vi "Maintenance.vi"() -> ()   [LabVIEW 2016, in "User Interface.lvlib"]
uses:
  User Interface.lvlib
  Maintenance command.ctl
  Database/Database.lvlib
  CAN/CAN.lvlib
  DAQ Hardware/DAQ Hardware.lvlib
  DAQ IO/DAQ IO.lvlib
  DC PWS/DC PWS.lvlib
  DMM/DMM.lvlib
  Func Generator/Func Generator.lvlib
  Oscilloscope/Oscilloscope.lvlib
  S-Matrix/S-Matrix.lvlib
  ARINC/ARINC.lvlib
  Maintenance Data highway.ctl
  Environment Chamber/Environment Chamber.lvlib
  VI Name.ctl
  CVT/CVT.lvlib
  DAQ Hardware/Timing AI DAQ Setting.ctl
  Instrument Address Command.ctl
  <vilib>/Utility/miscctls.llb/LVPointTypeDef.ctl
  Data Analysis/Data Analysis.lvlib
  Serial Hardware/Serial Hardware.lvlib
  <vilib>/NI/Current Value Table/Current Value Table.lvlib
  <vilib>/NI/Current Value Table/DataTypes/Boolean_Static Read.vi
  <vilib>/xnet/xnet.llb/XNET Frame Type CAN.ctl
  <vilib>/xnet/xnet.llb/XNET Frame CAN.ctl
panel:
  out "Analog Data":cluster{"DBL Array":dbl[]}[](graph)
  in  "Apply Command":bool
  out "Time 2":string="Authentication"
  in  "View Data":bool
  in  "Tab Control":T1(tab)
  in  "Channel Data":dbl[][](array[numeric])
  in  "DIO Apply Comm":bool
  in  "NI DAQ Command":enum16{"Acquire DI", "Stop DI"}(ring) caption="INPUT COMMAND"
  in  "NI DIO Connected":bool=TRUE
  in  "Sweep Spacing":enum16{"Linear", "Logarithmic"}(ring)
  in  "Unit (0: Vpp)":enum16{"Vpp", "Vrms", "dB"}(ring)
  in  "Sweep Time(Sec)":dbl step=0.05 format="%_4f"
  in  "Stop Freq(Hz)":dbl step=0.05 format="%_4f"
  in  "Start Freq(Hz)":dbl step=0.05 format="%_4f"
  in  "DC Offset (V)":dbl step=0.05 format="%_4f"
  in  "Amplitude":dbl step=0.05 format="%_4f"
  in  "Frequency(1000 Hz)":dbl step=0.05 format="%_4f"
  in  "Input Command":enum16{"Standad Waveform", "Frequency Sweep"}(ring)
  in  "FGen_Apply Command":bool
  in  "F.Gen Connected":bool=TRUE
  in  "Function":T2(ring)
  in  "Digital Output":T3
  in  "NI DAQ Control":T4={"NI DAQ Connected"=TRUE, "NI DAQ Command"=enum."Acquire AI", "AO Name"="AI 0", "AO Data In"=0.0, "Sampling rate"=5000.0, "Apply Command"=FALSE} {"Sampling rate" step=0.05; "AO Data In" step=0.05}
  in  "Digital Output":T5
  in  "DMM Control":T6={"DMM Connected"=TRUE, "Data Out"=0.0, "DMM Command"=enum."DC Voltage", "Apply Command"=FALSE, "Continuity"=FALSE} {"Data Out" step=0.05}
  out "Digital Input":T7
  out "Voltage(V)":dbl step=0.05 format="%2_4f"
  out "Current(A)":dbl step=0.05 format="%_4f"
  out "Data Out":dbl step=0.05
  in  "Data In":dbl step=0.05
  in  "DC Apply Command":bool
  in  "DC PWS Connected":bool=TRUE
  in  "DC PWS Command":T8(ring) caption="INPUT COMMAND"
  in  "Scope Apply Command":bool
  in  "Scope Channel":T9(ring) caption="Channel"
  in  "Scope Connected":bool=TRUE
  in  "Scope Command":T10(ring) caption="INPUT COMMAND"
  in  "Serial Command":T11(ring) caption="Measurement Command"
  in  "Serial Apply Command":bool
  in  "Command":string
  in  "Serial Connected":bool=TRUE
  out "CAN Monitor":string[][](table)
  in  "NI DAQ Connected":bool=TRUE
  in  "NI CAN Command":T12(ring)
  in  "Baud rate":dbl caption="Baudrate(Kbps)" step=0.05
  in  "CAN Command":bool
  in  "Interface Name":refnum<k21>
  in  "CAN Frame":T13[](array[typedef])=[{"timestamp"=timestamp(0 s since 1904-01-01), "payload"=[1, 2, 3, 4, 5, 6, 7, 8], "identifier"=2, "type"=0, "extended?"=FALSE, "echo?"=FALSE}, {"timestamp"=timestamp(0 s since 1904-01-01), "payload"=[0, 1, 2, 3, 4, 5, 6, 7], "identifier"=3, "type"=0, "extended?"=FALSE, "echo?"=FALSE}] {"payload" format="%x"; "timestamp" format="%<%.7X\n%x>T"; "type" items=["CAN Data"=0, "CAN Remote"=1, "CAN Bus Error"=2, "CAN 2.0 Data"=8, "CAN FD Data"=16, "CAN FD+BRS Data"=24, "J1939 Data"=192, "Delay"=224, "Log Trigger"=225, "Start Trigger"=226]; "identifier" format="%x"}
  out "CAN Monitor":string[][](table)
  out "Humidity":dbl step=0.05 format="%.2g"
  out "Temperature":dbl step=0.05 format="%.2g"
  out "Program State":T15 {"Remaining Counter B" step=0.05 format="%.2g"; "Remaining Counter A" step=0.05 format="%.2g"; "Remaining Time" step=0.05 format="%.2g"; "Humi Set Point" step=0.05 format="%.2g"; "Temp Set Point" step=0.05 format="%.2g"; "Step No" step=0.05 format="%.2g"; "Program No" step=0.05 format="%.2g"}
  in  "Meas Command":T16(ring) caption="Measurement Command"
  in  "ESPEC Apply Command":bool
  in  "ESPEC Connected":bool=TRUE
  in  "Exit":bool
  in  "DAQ Type":enum16{"Hardware", "Simulation"}(ring)=enum."Simulation"
  out "Fetch?":bool
  out "error out":errorcluster
  in  "error in (no error)":errorcluster
  # "NI CAN"
  # "NI 6363 DIO"
  # "NI 6515 Digital Input"
  # "NI 6515 Digital Output"
  # "Serial Inst Control"
  # "Scope Control"
  # "NI DIO(6515) Control"
  # "Function Generator Control"
  # "NI DAQ(6363) Control"
  # "DMM Control"
  # "DC Control"
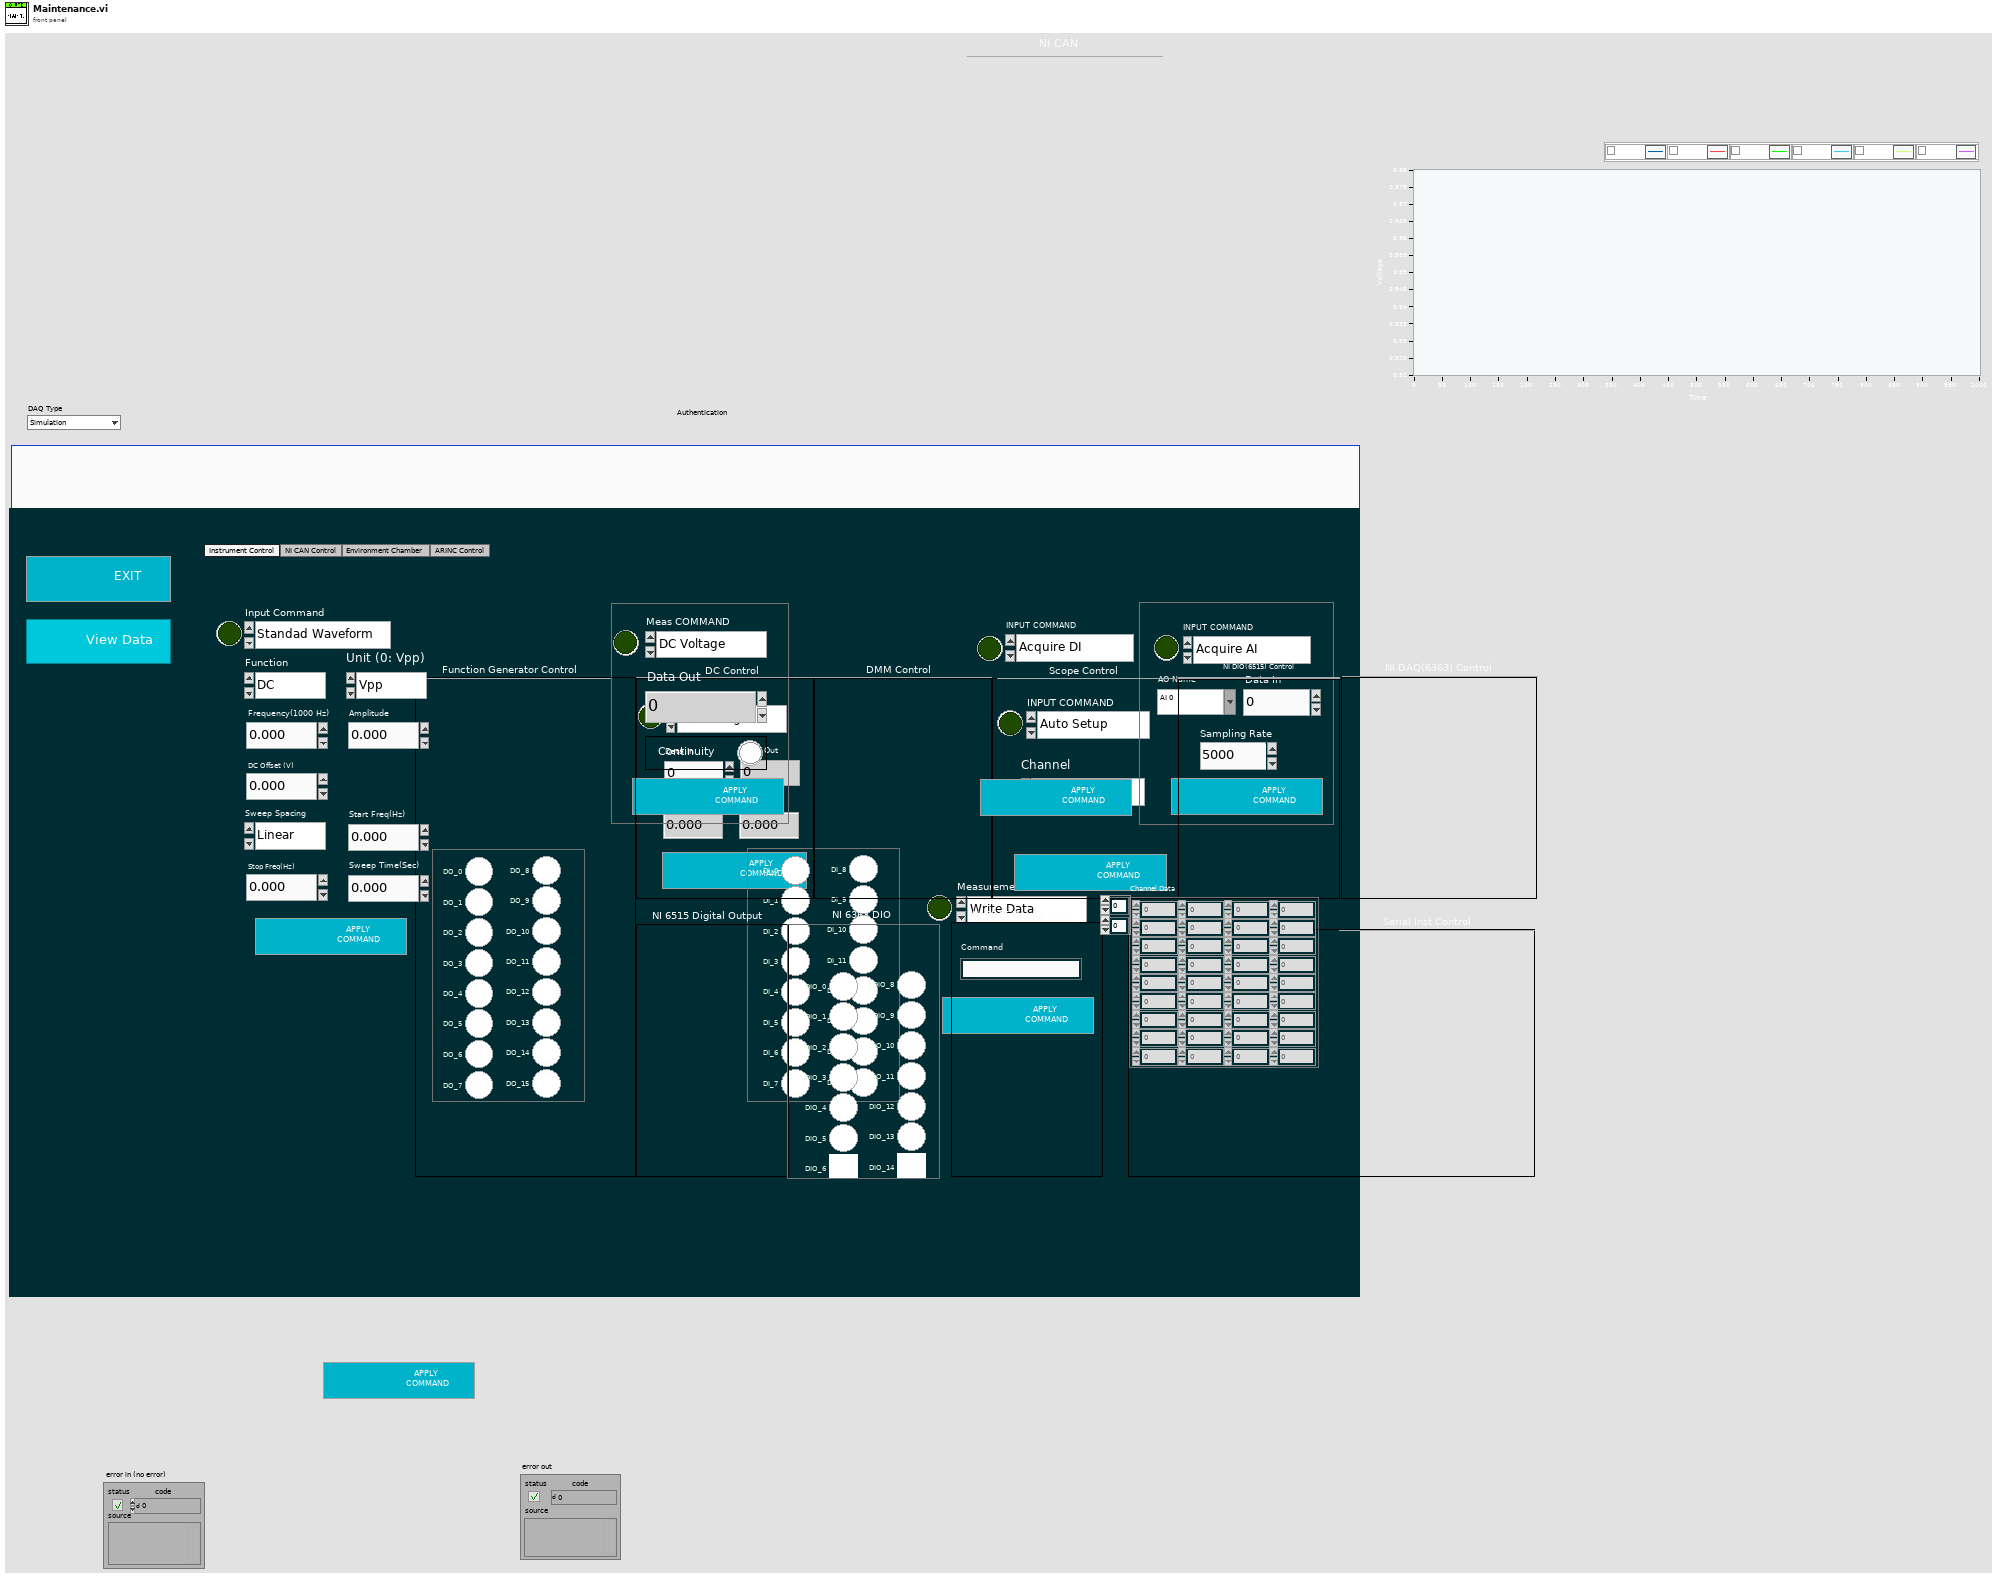
[diagram p1: front panel]
types:
  T1 = enum32{"Instrument Control", "NI CAN Control", "Environment Chamber", "ARINC Control"}
  T2 = enum16{"DC", "Sine", "Square", "Triangle", "Ramp", "Pulse", "Noise"}
  T3 = cluster{"DIO_0":bool, "DIO_1":bool, "DIO_2":bool, "DIO_3":bool, "DIO_4":bool, "DIO_5":bool, "DIO_6":bool, "DIO_7":bool, "DIO_8":bool, "DIO_9":bool, "DIO_10":bool, "DIO_11":bool, "DIO_12":bool, "DIO_13":bool, "DIO_14":bool, "DIO_15":bool}
  T4 = cluster{"NI DAQ Connected":bool, "NI DAQ Command":enum16{"Acquire AI", "Log Data", "Stop Log Data", "Stop AI", "Acquire DI", "Stop DI", "Update Rate", "Write AO"}, "AO Name":string, "AO Data In":dbl, "Sampling rate":dbl, "Apply Command":bool}
  T5 = cluster{"DO_0":bool, "DO_1":bool, "DO_2":bool, "DO_3":bool, "DO_4":bool, "DO_5":bool, "DO_6":bool, "DO_7":bool, "DO_8":bool, "DO_9":bool, "DO_10":bool, "DO_11":bool, "DO_12":bool, "DO_13":bool, "DO_14":bool, "DO_15":bool}
  T6 = cluster{"DMM Connected":bool, "Data Out":dbl, "DMM Command":enum16{"DC Voltage", "AC Voltage", "2 Wire Resistance", "Continuity"}, "Apply Command":bool, "Continuity":bool}
  T7 = cluster{"DI_0":bool, "DI_1":bool, "DI_2":bool, "DI_3":bool, "DI_4":bool, "DI_5":bool, "DI_6":bool, "DI_7":bool, "DI_8":bool, "DI_9":bool, "DI_10":bool, "DI_11":bool, "DI_12":bool, "DI_13":bool, "DI_14":bool, "DI_15":bool}
  T8 = enum16{"Set Voltage", "Set Current", "Set Power", "DC Parameter", "Measure Current", "Measure Voltage", "Output"}
  T9 = enum16{"Channel 1", "Channel 2", "Channel 3", "Channel 4"}
  T10 = enum16{"Auto Setup", "Config Channel", "Config DVM", "Acquire Waveform"}
  T11 = enum16{"Write Data", "Acquire Data", "Start Logging", "Stop Logging"}
  T12 = enum16{"Read CAN Data", "Write CAN Data", "Set Baudrate", "Start Logging Data", "Stop Logging Data"}
  T13 = typedef "XNET Frame CAN.ctl" = cluster{"timestamp":timestamp, "payload":u8[], "identifier":u32, "type":T14, "extended?":bool, "echo?":bool}
  T14 = typedef "XNET Frame Type CAN.ctl" = u8
  T15 = cluster{"Program No":dbl, "Step No":dbl, "Temp Set Point":dbl, "Humi Set Point":dbl, "Remaining Time":dbl, "Remaining Counter A":dbl, "Remaining Counter B":dbl}
  T16 = enum16{"Output On", "Output Off", "Acquire Data", "Start Log Data", "Stop Log Data", "Program Status"}
  T17 = typedef "LVPointTypeDef.ctl" = cluster{"Horizontal":i16, "Vertical":i16}
  T18 = typedef "User Interface.lvlib/Maintenance Data highway.ctl" = cluster{"Connection?":cluster{"DC PWS ?":bool, "DMM ?":bool, "FGEN ?":bool, "Oscill ?":bool, "NI DAQ ?":bool, "NI DIO ?":bool, "NI CAN ?":bool, "ESPEC ?":bool, "ARINC ?":bool, "MATRIX ?":bool}, "Inst Connected":refnum<vi>[], "Signal Name":cluster{"AI":string[], "AO":string[], "DI":string[], "DO":string[]}}
  T19 = typedef "User Interface.lvlib/Maintenance command.ctl" = enum16{"Init", "Main", "Close"}
  T20 = typedef "Current Value Table.lvlib/Group Data.ctl" = cluster{"Double":dbl[], "Single":sgl[], "I64":i64[], "I32":i32[], "I16":i16[], "I8":i8[], "U64":u64[], "U32":u32[], "U16":u16[], "U8":u8[], "String":string[], "Boolean":bool[], "Array of U8":cluster{"U8 Array":u8[]}[], "Array of U16":cluster{"U16 Array":u16[]}[], "Array of U32":cluster{"U32 Array":u32[]}[], "Array of U64":cluster{"U64 Array":u64[]}[], "Array of I64":cluster{"I64 Array":i64[]}[], "Array of I32":cluster{"I32 Array":i32[]}[], "Array of I16":cluster{"I16 Array":i16[]}[], "Array of I8":cluster{"I8 Array":i8[]}[], "Array of Double":cluster{"DBL Array":dbl[]}[], "Array of Single":cluster{"SGL Array":sgl[]}[], "Array of Boolean":cluster{"Boolean Array":bool[]}[], "Array of String":cluster{"String Array":string[]}[]}
  T21 = cluster{"Double[0]":dbl, "Double[1]":dbl, "Double[2]":dbl, "Double[3]":dbl, "Double[4]":dbl, "Double[5]":dbl, "Double[6]":dbl}
  T22 = cluster{"Boolean[0]":bool, "Boolean[1]":bool, "Boolean[2]":bool, "Boolean[3]":bool, "Boolean[4]":bool, "Boolean[5]":bool, "Boolean[6]":bool, "Boolean[7]":bool, "Boolean[8]":bool, "Boolean[9]":bool, "Boolean[10]":bool, "Boolean[11]":bool, "Boolean[12]":bool, "Boolean[13]":bool, "Boolean[14]":bool, "Boolean[15]":bool}
  T23 = typedef "User Interface.lvlib/Instrument Address Command.ctl" = enum16{"Init", "Read", "Write", "Close"}
  T24 = cluster{"Address":dbl, "Voltage Level":dbl, "Enable Output":bool}
  T25 = cluster{"Meas Command":enum16{"Voltage", "Current", "Power"}, "Address":dbl}
  T26 = cluster{"Waveform Function (1: Sine)":u16, "Frequency (1000 Hz)":dbl, "Amplitude (1)":dbl, "Unit (0: Vpp)":u16, "DC Offset (0.00 V)":dbl}
  T27 = cluster{"Sweep Spacing (0: Linear)":u16, "Sweep Time (1.00 s)":dbl, "Stop  Frequency (1000.0 Hz)":dbl, "Start Frequency (100.0 Hz)":dbl, "Enable/Disable Freq Sweep":bool}
  T28 = cluster{"Channel Name (0: Channel 1)":i32, "Coupling (1: DC)":i32, "Vertical Offset (0.0)":dbl, "Vertical Range (40.0 V)":dbl, "Probe Attenuation (1.0)":dbl, "Enable Channel (T: Enable)":bool, "Impedance (0: 1 MOhm)":i32, "Vertical Scale (5.0 V)":dbl, "Vertical Setting (1: Vertical Range)":i32}
  T29 = typedef "DAQ Hardware.lvlib/Timing AI DAQ Setting.ctl" = cluster{"rate":dbl, "samples per channel":i32, "sample mode":i32}
  T30 = typedef "User Interface.lvlib/VI Name.ctl" = enum16{"Dashboard", "Maintenance", "Recipe", "Inst Calibration", "Testing", "Report"}
  T31 = cluster{"[0]":bool, "[1]":bool, "[2]":bool, "[3]":bool, "[4]":bool, "[5]":bool, "[6]":bool, "[7]":bool, "[8]":bool, "[9]":bool}
  T32 = enum16{"DC Voltage", "AC Voltage", "2 Wire Resistance", "Continuity"}
  T33 = enum16{"Acquire AI", "Log Data", "Stop Log Data", "Stop AI", "Acquire DI", "Stop DI", "Update Rate", "Write AO"}
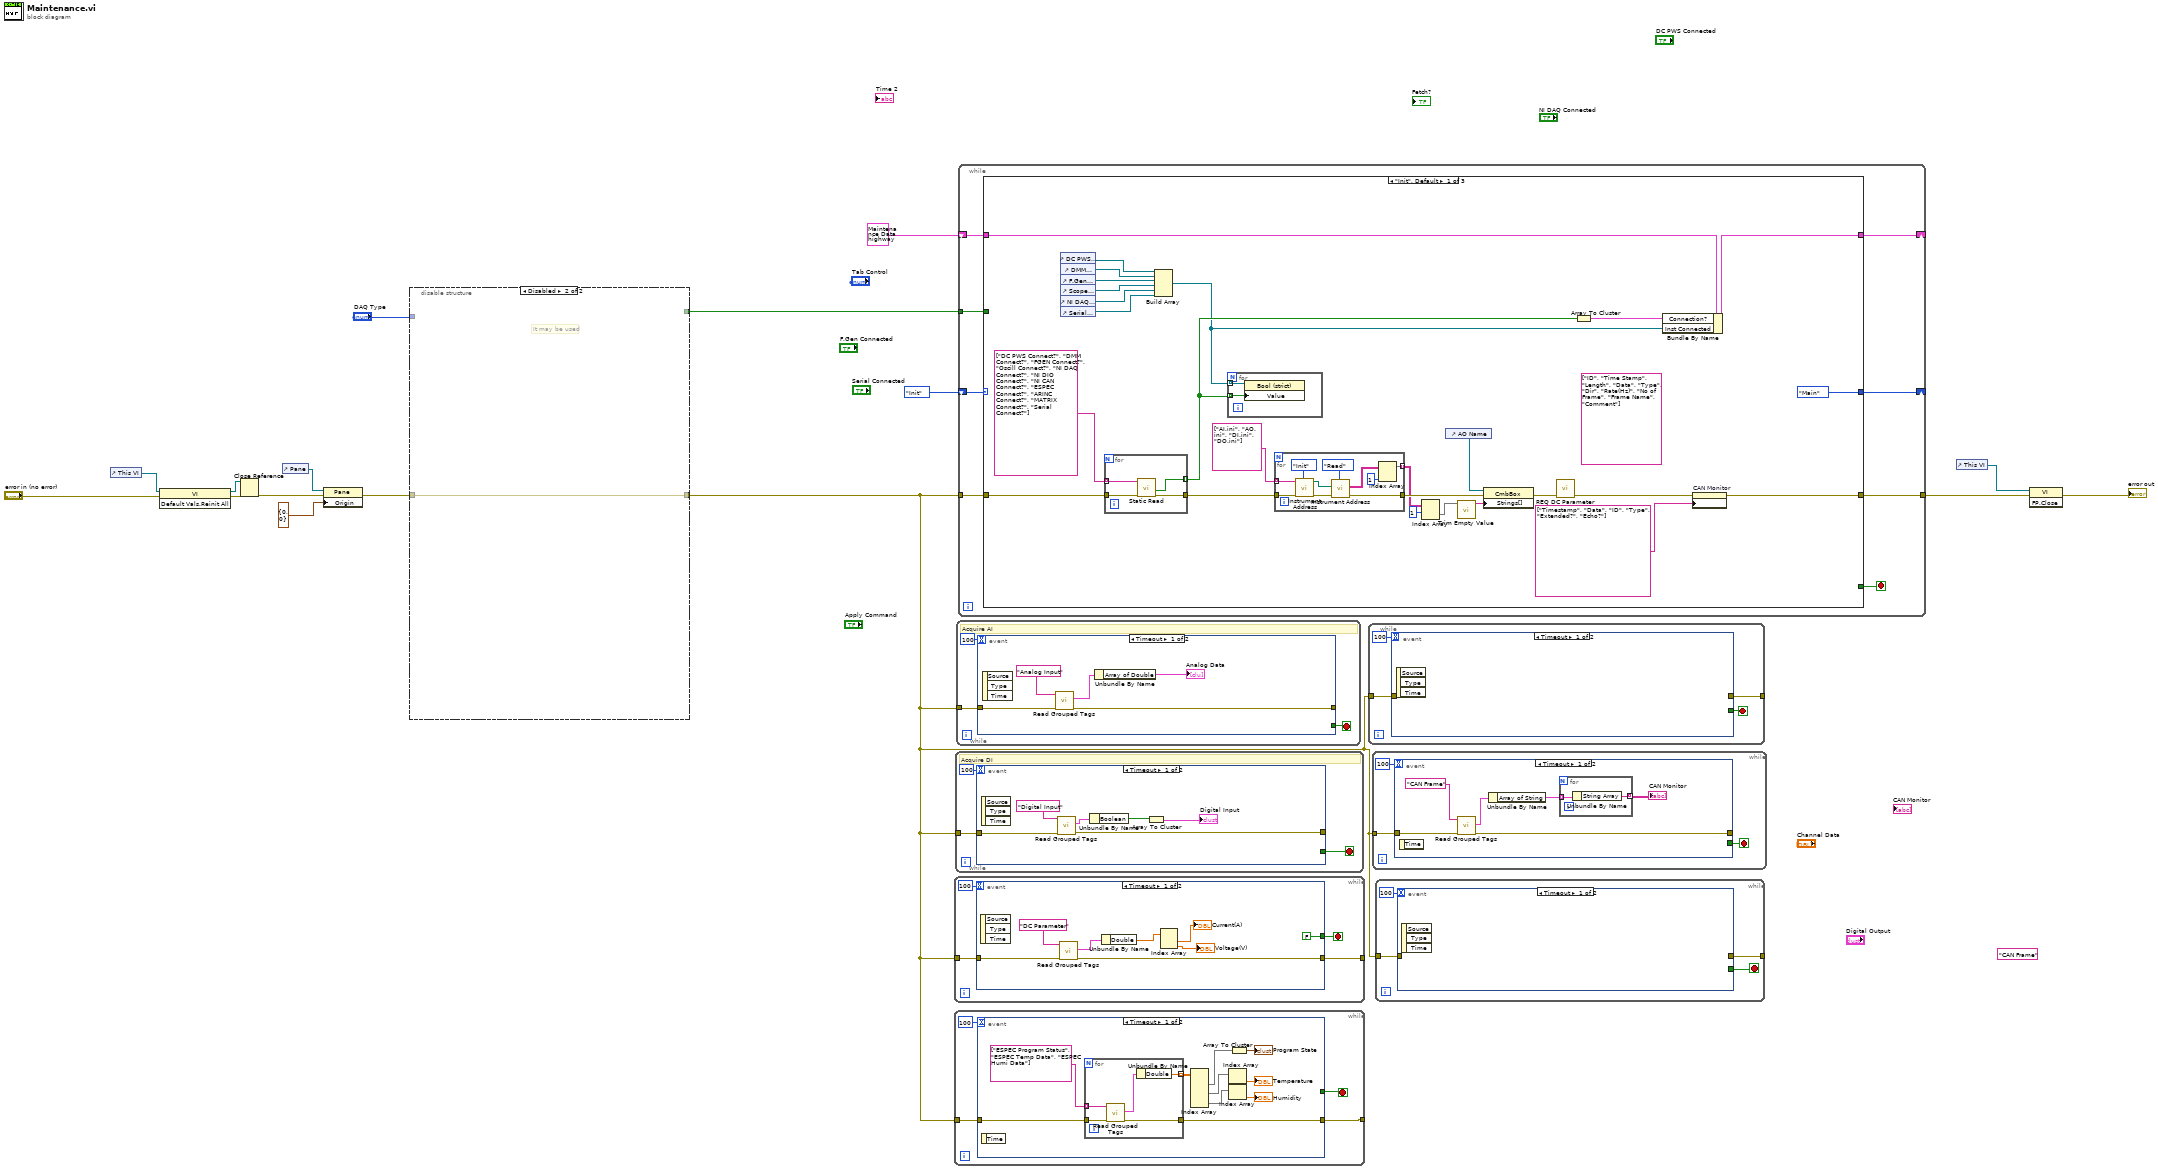
[diagram p0: block diagram]
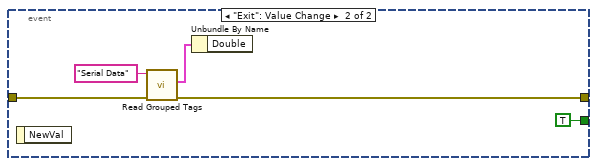
[diagram p2: hidden frame]
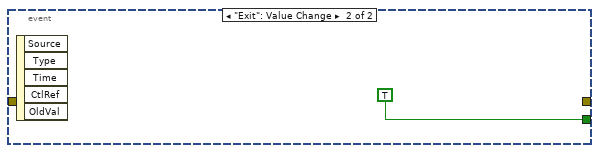
[diagram p3: hidden frame]
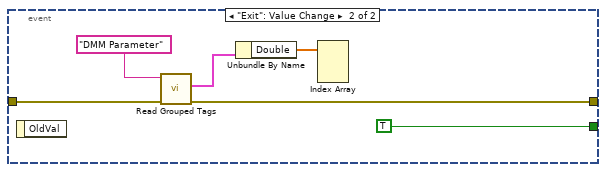
[diagram p4: hidden frame]
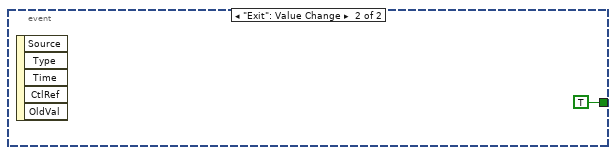
[diagram p5: hidden frame]
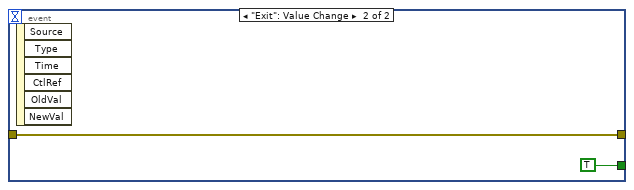
[diagram p6: hidden frame]
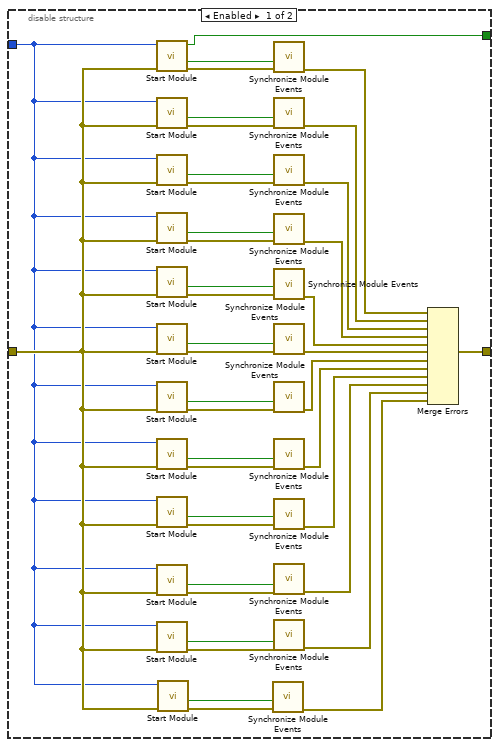
[diagram p7: hidden frame]
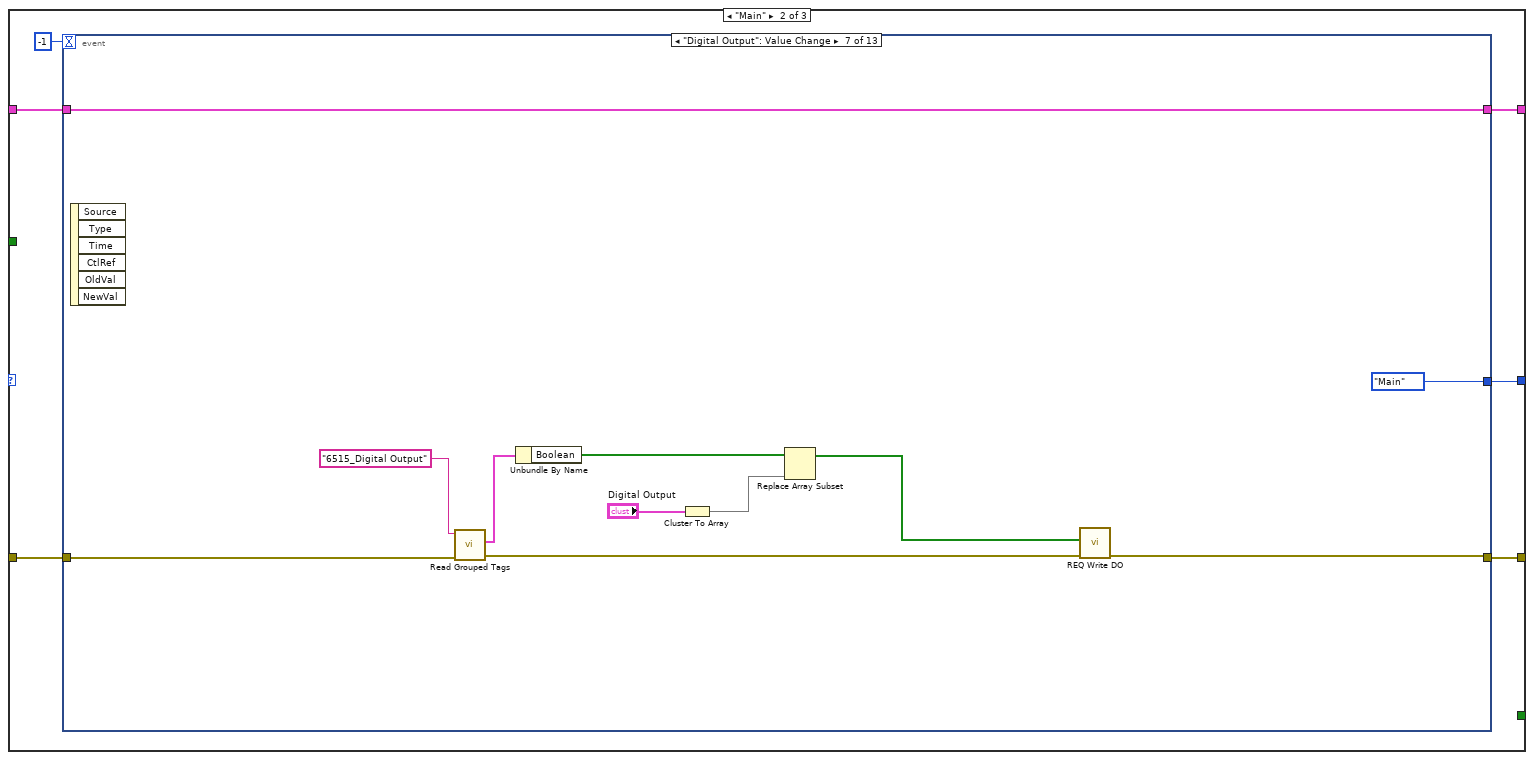
[diagram p8: hidden frame]
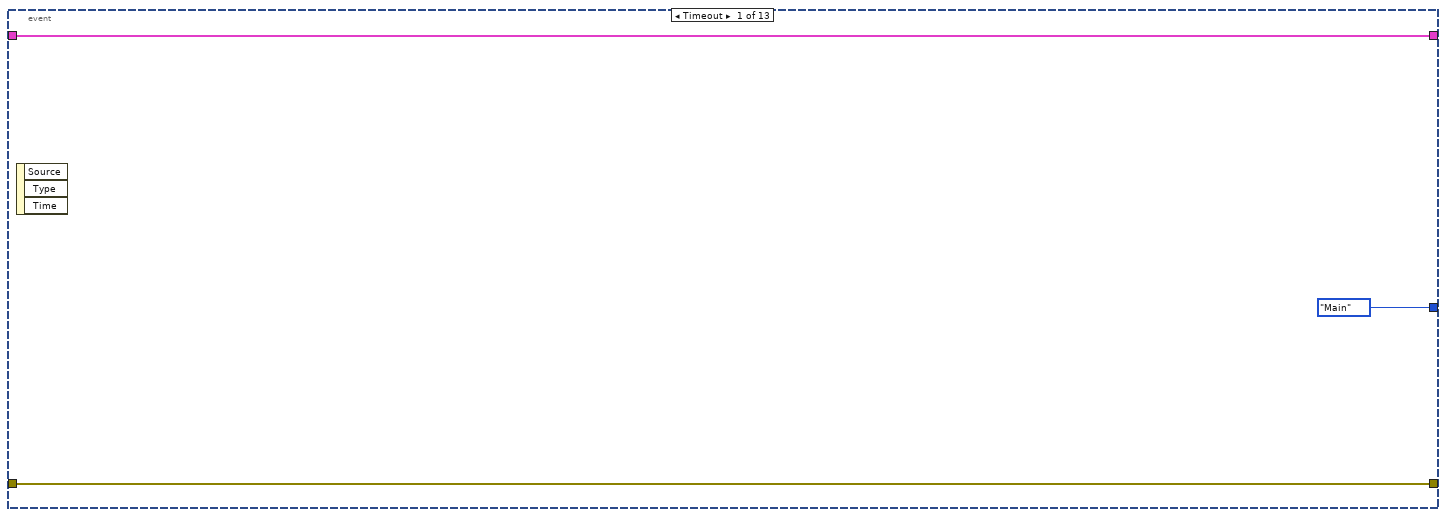
[diagram p9: hidden frame]
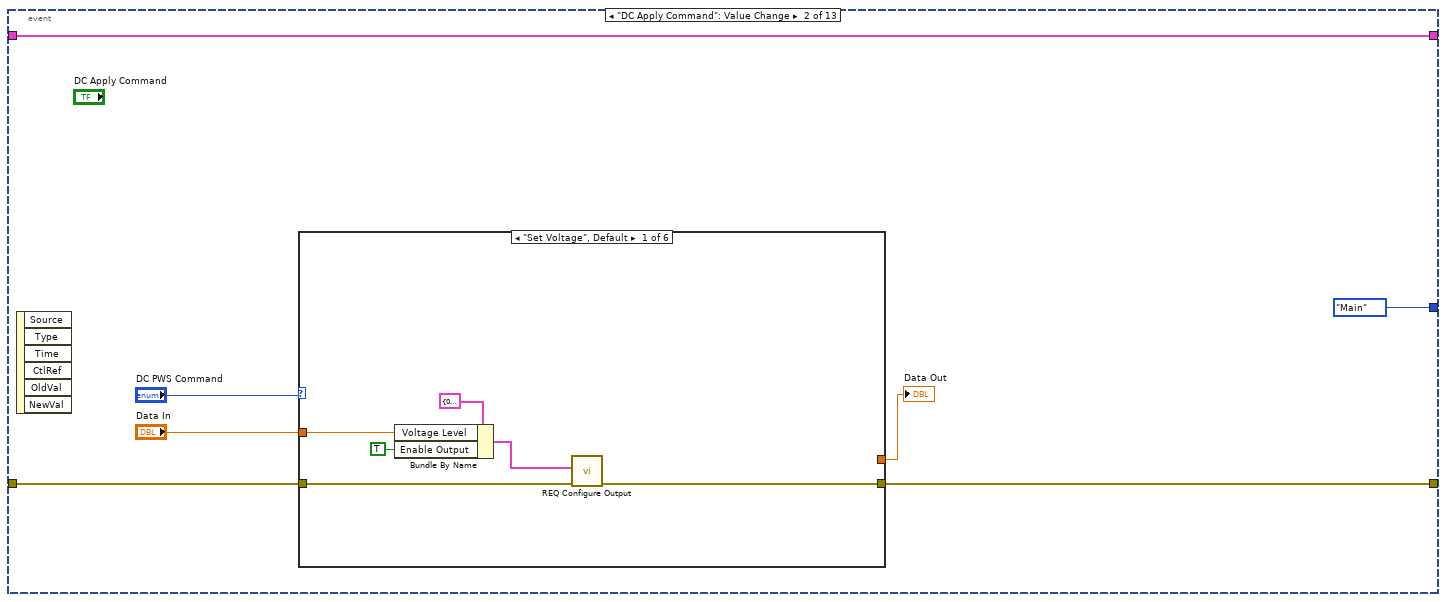
[diagram p10: hidden frame]
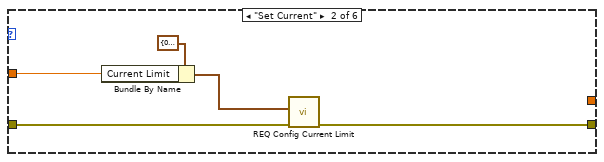
[diagram p11: hidden frame]
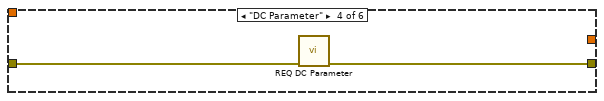
[diagram p13: hidden frame]
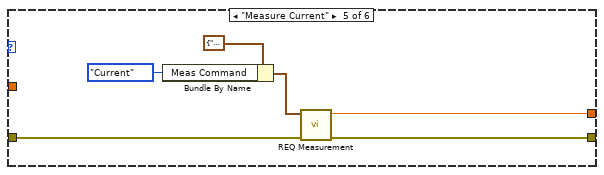
[diagram p14: hidden frame]
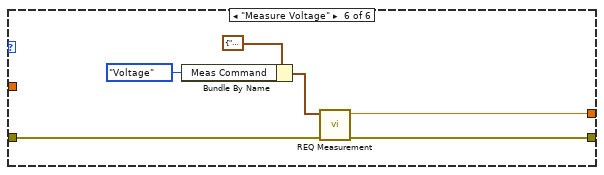
[diagram p15: hidden frame]
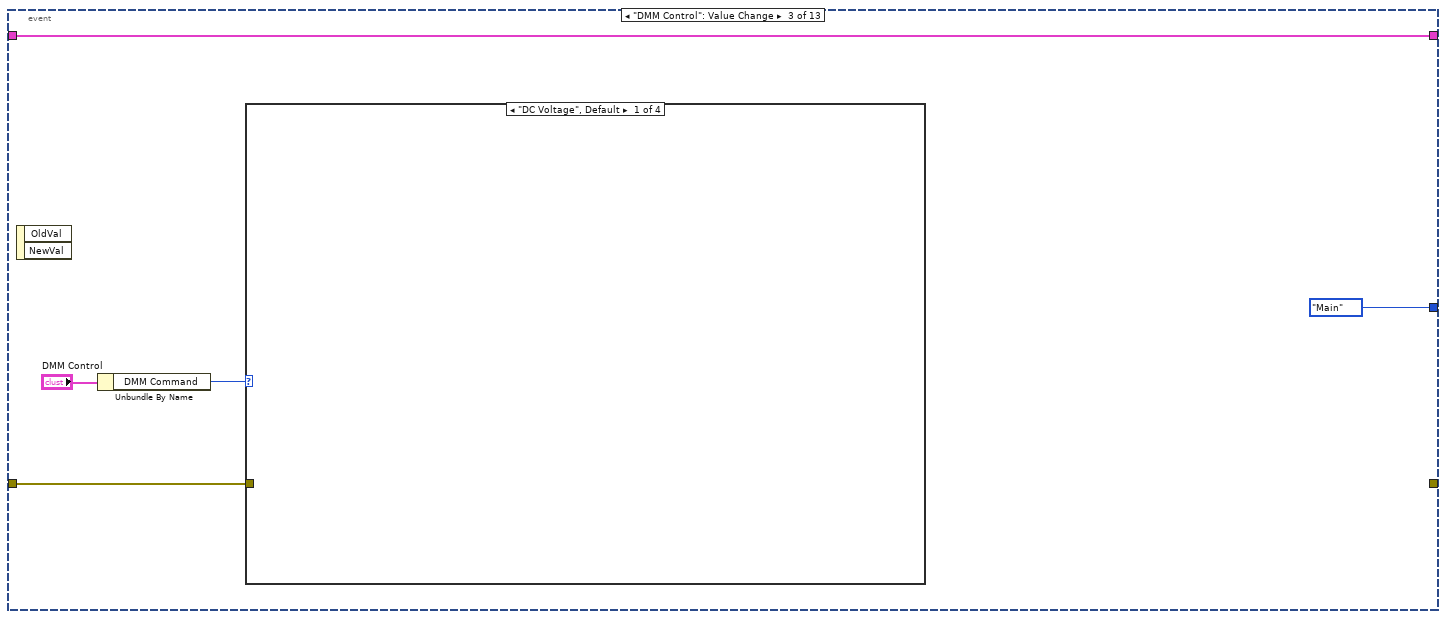
[diagram p16: hidden frame]
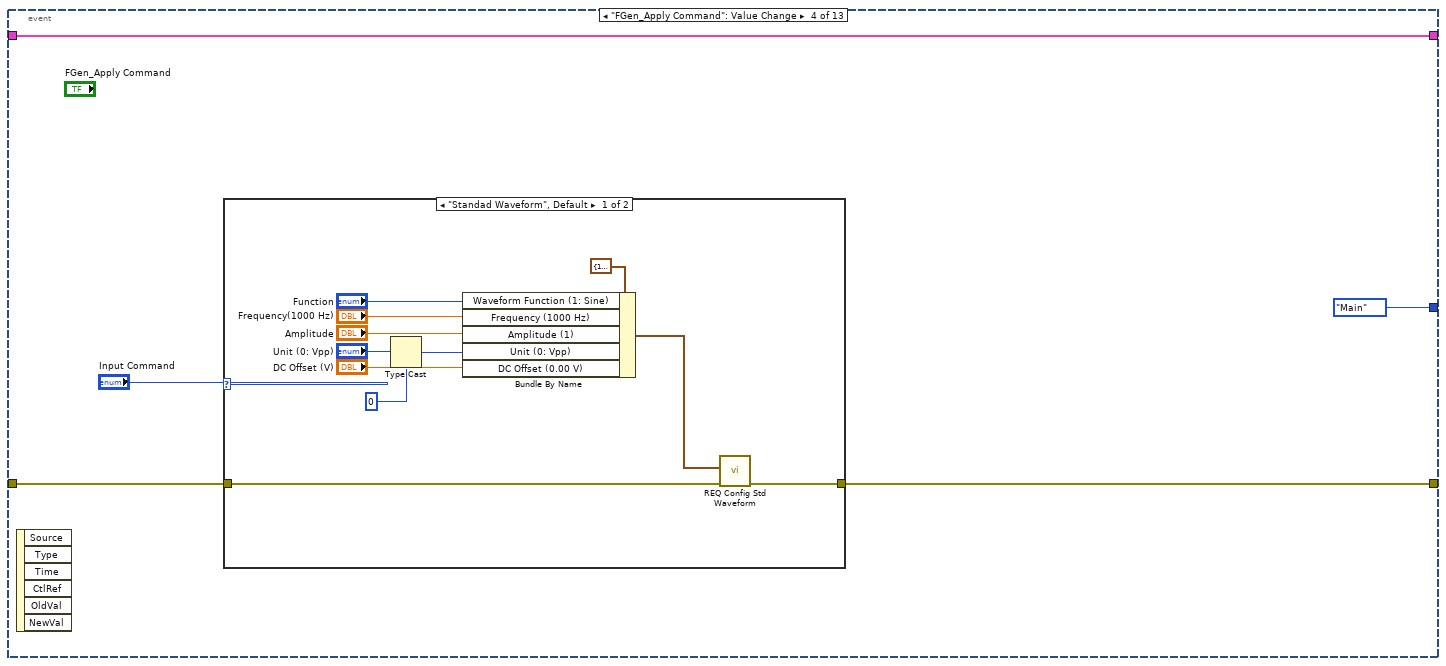
[diagram p20: hidden frame]
diagram:
  (unwired) "CAN Frame" ("Group")
  n1 = control-ref of="This VI"() -> (w12:refnum<vi>)
  n2 = invoke class="VI" method="Default Vals.Reinit All"(reference=w12, error in="error in (no error)") -> (reference out=w10:refnum<vi>, error out=w11:errorcluster)  [unwired: 1 in, 1 out]
  n3 = Close Reference(reference=w10, error in (no error)=w11) -> (error out=w9:errorcluster)
  n4 = control-ref of="Pane"() -> (w16:refnum<vi>)
  n5 = property class="Pane"(reference=w16, error in=w9, "Origin"=T17 {"Horizontal"=0, "Vertical"=0}) -> (error out=w4:errorcluster)  [unwired: 1 out]
  n6 = disable-structure shown="Disabled" {
    disable-tunnel: [w29 w57] -> w1
    disable-tunnel: [w28 _] -> w14
    disable-tunnel: w4 -> [w20 w57]
    disable-tunnel: "DAQ Type" -> [w19 _]
    frame Enabled {
      n7 = call "Start Module.vi"("error in"=w20, "DAQ Type"=w19) -> ("error out"=w23:errorcluster, "Wait for Event Sync?"=w22:bool, "Module Was Already Running?"=w28:bool)  [unwired: 6 in, 1 out]
      n8 = call "Start Module.vi"("error in"=w20, "DAQ Type"=w19) -> ("error out"=w49:errorcluster, "Wait for Event Sync?"=w47:bool)  [unwired: 6 in, 2 out]
      n9 = call "Start Module.vi"("error in"=w20, "DAQ Type"=w19) -> ("error out"=w50:errorcluster, "Wait for Event Sync?"=w46:bool)  [unwired: 6 in, 2 out]
      n10 = call "Start Module.vi"("error in"=w20, "DAQ Type"=w19) -> ("error out"=w48:errorcluster, "Wait for Event Sync?"=w45:bool)  [unwired: 6 in, 2 out]
      n11 = call "Start Module.vi"("error in"=w20, "DAQ Type"=w19) -> ("error out"=w51:errorcluster, "Wait for Event Sync?"=w44:bool)  [unwired: 6 in, 2 out]
      n12 = call "Start Module.vi"("error in"=w20, "DAQ Type"=w19) -> ("error out"=w52:errorcluster, "Wait for Event Sync?"=w43:bool)  [unwired: 6 in, 2 out]
      n13 = call "Start Module.vi"("error in"=w20, "DAQ Type"=w19) -> ("error out"=w53:errorcluster, "Wait for Event Sync?"=w42:bool)  [unwired: 6 in, 2 out]
      n14 = call "Start Module.vi"("error in"=w20, "DAQ Type"=w19) -> ("error out"=w54:errorcluster, "Wait for Event Sync?"=w41:bool)  [unwired: 6 in, 2 out]
      n15 = call "Start Module.vi"("error in"=w20, "DAQ Type"=w19) -> ("error out"=w55:errorcluster, "Wait for Event Sync?"=w40:bool)  [unwired: 6 in, 2 out]
      n16 = call "Start Module.vi"("error in"=w20, "DAQ Type"=w19) -> ("error out"=w56:errorcluster, "Wait for Event Sync?"=w39:bool)  [unwired: 6 in, 2 out]
      n17 = call "Start Module.vi"("error in"=w20, "DAQ Type"=w19) -> ("error out"=w26:errorcluster, "Wait for Event Sync?"=w25:bool)  [unwired: 6 in, 2 out]
      n18 = call "Start Module.vi"("error in"=w20, "DAQ Type"=w19) -> ("error out"=w21:errorcluster, "Wait for Event Sync?"=w18:bool)  [unwired: 6 in, 2 out]
      n19 = call "Synchronize Module Events.vi"("error in"=w21, "Wait for Event Sync?"=w18) -> ("error out"=w17:errorcluster)  [unwired: 9 in]
      n20 = call "Synchronize Module Events.vi"("error in"=w23, "Wait for Event Sync?"=w22) -> ("error out"=w38:errorcluster)  [unwired: 9 in]
      n21 = call "Synchronize Module Events.vi"("error in"=w49, "Wait for Event Sync?"=w47) -> ("error out"=w37:errorcluster)  [unwired: 9 in]
      n22 = call "Synchronize Module Events.vi"("error in"=w50, "Wait for Event Sync?"=w46) -> ("error out"=w36:errorcluster)  [unwired: 9 in]
      n23 = call "Synchronize Module Events.vi"("error in"=w48, "Wait for Event Sync?"=w45) -> ("error out"=w27:errorcluster)  [unwired: 9 in]
      n24 = call "Synchronize Module Events.vi"("error in"=w51, "Wait for Event Sync?"=w44) -> ("error out"=w35:errorcluster)  [unwired: 9 in]
      n25 = call "Synchronize Module Events.vi"("error in"=w52, "Wait for Event Sync?"=w43) -> ("error out"=w34:errorcluster)  [unwired: 9 in]
      n26 = call "Synchronize Module Events.vi"("error in"=w53, "Wait for Event Sync?"=w42) -> ("error out"=w33:errorcluster)  [unwired: 9 in]
      n27 = call "Synchronize Module Events.vi"("error in"=w54, "Wait for Event Sync?"=w41) -> ("error out"=w32:errorcluster)  [unwired: 9 in]
      n28 = call "Synchronize Module Events.vi"("error in"=w55, "Wait for Event Sync?"=w40) -> ("error out"=w31:errorcluster)  [unwired: 9 in]
      n29 = call "Synchronize Module Events.vi"("error in"=w56, "Wait for Event Sync?"=w39) -> ("error out"=w30:errorcluster)  [unwired: 9 in]
      n30 = call "Synchronize Module Events.vi"("error in"=w26, "Wait for Event Sync?"=w25) -> ("error out"=w24:errorcluster)  [unwired: 9 in]
      n31 = Merge Errors(w38, w37, w36, w27, w35, w34, w33, w32, w31, w30, w24, w17) -> (w29:errorcluster)
    }
    frame Disabled {
      # "It may be used"
    }
  }
  n32 = while {
    tunnel: w1 -> [w60]
    tunnel: [w59] -> _
    stop <- w61 stop-if-true
    n33 = event shown="[0] Timeout" {
      selector: _ -> [_ _]
      dyn-events: _ -> [_ _]
      timeout: 100 -> [_ _]
      tunnel: [FALSE TRUE] -> w61
      tunnel: w60 -> [w66 w70]
      tunnel: [w62 w70] -> w59
      event Timeout {
        n34 = event-data() -> ()  [unwired: 1 in, 3 out]
        n35 = call <vilib>:"Read Grouped Tags.vi"("error in (no error)"=w66, "Group"="DC Parameter") -> ("error out"=w62:errorcluster, "Data"=w67:T20)  [unwired: 8 in]
        n36 = Unbundle By Name(w67) -> ("Double"=w65:dbl[])
        n37 = Index Array(array=w65) -> (element #1=→"Current(A)":dbl, element #2=→"Voltage(V)":dbl)  [unwired: 2 in]
      }
      event "Exit": Value Change {
        n38 = event-data() -> ()  [unwired: 1 in, 1 out]
      }
    }
  }
  n39 = while {
    tunnel: w1 -> [w73]
    tunnel: [w72] -> _
    stop <- w75 stop-if-true
    n40 = event shown="[0] Timeout" {
      selector: _ -> [_ _]
      dyn-events: _ -> [_ _]
      timeout: 100 -> [_ _]
      tunnel: [_ TRUE] -> w75
      tunnel: w73 -> [w85 _]
      tunnel: [w84 _] -> w72
      event Timeout {
        n41 = event-data() -> ()  [unwired: 1 in, 1 out]
        n42 = for {
          tunnel: w85 -> [w90]
          tunnel: [w89] -> w84
          tunnel: string[] ["ESPEC Program Status", "ESPEC Temp Data", "ESPEC Humi Data"] -> [w88] mode=indexing
          tunnel: [w86] -> w81 mode=indexing
          n43 = call <vilib>:"Read Grouped Tags.vi"("error in (no error)"=w90, "Group"=w88) -> ("error out"=w89:errorcluster, "Data"=w87:T20)  [unwired: 8 in]
          n44 = Unbundle By Name(w87) -> ("Double"=w86:dbl[])
        }
        n45 = Index Array(array=w81) -> (element #1=w80:dbl[], element #2=w79:dbl[], element #3=w78:dbl[])  [unwired: 6 in]
        n46 = Index Array(array=w79) -> (element=→"Temperature":dbl)  [unwired: 1 in]
        n47 = Index Array(array=w78) -> (element=→"Humidity":dbl)  [unwired: 1 in]
        n48 = Array To Cluster(array=w80) -> (cluster=→"Program State":T21)
      }
      event "Exit": Value Change {
        n49 = event-data() -> ()  [unwired: 1 in, 5 out]
      }
    }
  }
  n50 = while {
    tunnel: w1 -> [w94]
    stop <- w92 stop-if-true
    # "Acquire DI"
    n51 = event shown="[0] Timeout" {
      selector: _ -> [_ _]
      dyn-events: _ -> [_ _]
      timeout: 100 -> [_ _]
      tunnel: w94 -> [w99 w101]
      tunnel: [w96 w101] -> _
      tunnel: [_ TRUE] -> w92
      event Timeout {
        n52 = event-data() -> ()  [unwired: 1 in, 3 out]
        n53 = call <vilib>:"Read Grouped Tags.vi"("error in (no error)"=w99, "Group"="Digital Input") -> ("error out"=w96:errorcluster, "Data"=w98:T20)  [unwired: 8 in]
        n54 = Unbundle By Name(w98) -> ("Boolean"=w97:bool[])
        n55 = Array To Cluster(array=w97) -> (cluster=→"Digital Input":T22)
      }
      event "Exit": Value Change {
        n56 = event-data() -> ()  [unwired: 1 in, 6 out]
      }
    }
  }
  n57 = while {
    tunnel: w1 -> [w103]
    stop <- w105 stop-if-true
    # "Acquire AI"
    n58 = event shown="[0] Timeout" {
      selector: _ -> [_ _]
      dyn-events: _ -> [_ _]
      timeout: 100 -> [_ _]
      tunnel: [_ TRUE] -> w105
      tunnel: w103 -> [w108 w111]
      tunnel: [w107 w111] -> _
      event Timeout {
        n59 = event-data() -> ()  [unwired: 1 in, 3 out]
        n60 = call <vilib>:"Read Grouped Tags.vi"("error in (no error)"=w108, "Group"="Analog Input") -> ("error out"=w107:errorcluster, "Data"=w110:T20)  [unwired: 8 in]
        n61 = Unbundle By Name(w110) -> ("Array of Double"=→"Analog Data":cluster{"DBL Array":dbl[]}[])
      }
      event "Exit": Value Change {
        n62 = event-data() -> ()  [unwired: 1 in, 6 out]
      }
    }
  }
  n63 = while {
    shift-right: [w118] -> _
    shift-left: Maintenance_command."Init" -> [w120]
    tunnel: w1 -> [w119]
    tunnel: w14 -> [w116]
    shift-right: [w114] -> _
    shift-left: T18 {"Connection?"={"DC PWS ?"=FALSE, "DMM ?"=FALSE, "FGEN ?"=FALSE, "Oscill ?"=FALSE, "NI DAQ ?"=FALSE, "NI DIO ?"=FALSE, "NI CAN ?"=FALSE, "ESPEC ?"=FALSE, "ARINC ?"=FALSE, "MATRIX ?"=FALSE}, "Inst Connected"=[], "Signal Name"={"AI"=[], "AO"=[], "DI"=[], "DO"=[]}} -> [w115]
    tunnel: [w113] -> w5
    stop <- w117 stop-if-true
    n64 = case shown="\"Init\", Default" w120 {
      tunnel: w119 -> [w143 w167 w383]
      tunnel: [Maintenance_command."Main" w164 Maintenance_command."Close"] -> w118
      tunnel: [_ _ TRUE] -> w117
      tunnel: w116 -> [_ _ w382]
      tunnel: w115 -> [w145 w166 w384]
      tunnel: [w142 w165 w384] -> w114
      tunnel: [w122 w163 w376] -> w113
      frame "Init", Default {
        (unwired) string[] ["ID", "Time Stamp", "Length", "Data", "Type", "Dir", "Rate(Hz)", "No of Frame", "Frame Name", "Comment"] ("Row Header Strings[]")
        n65 = control-ref of="DC PWS Connected"() -> (w140:refnum<vi>)
        n66 = control-ref of="DMM Connected"() -> (w139:refnum<vi>)
        n67 = control-ref of="F.Gen Connected"() -> (w138:refnum<vi>)
        n68 = control-ref of="Scope Connected"() -> (w137:refnum<vi>)
        n69 = control-ref of="NI DAQ Connected"() -> (w136:refnum<vi>)
        n70 = control-ref of="Serial Connected"() -> (w121:refnum<vi>)
        n71 = for {
          tunnel: string[] ["DC PWS Connect?", "DMM Connect?", "FGEN Connect?", "Oscill Connect?", "NI DAQ Connect?", "NI DIO Connect?", "NI CAN Connect?", "ESPEC Connect?", "ARINC Connect?", "MATRIX Connect?", "Serial Connect?"] -> [w162] mode=indexing
          tunnel: [w161] -> w135 mode=indexing
          tunnel: w143 -> [w160]
          tunnel: [w159] -> w134
          n72 = call-poly <vilib>:"Static Read.vi"("error in (no error)"=w160, "Tag Name"=w162) -> ("error out"=w159:errorcluster, "Value"=w161:bool)  [unwired: 8 in]
        }
        n73 = Build Array(w140, w139, w138, w137, w136, w121) -> (w125:refnum<vi>[])
        n74 = for {
          tunnel: w125 -> [w158] mode=indexing
          tunnel: w135 -> [w157] mode=indexing
          n75 = property class="Bool (strict)"(reference=w158, "Value"=w157) -> ()  [unwired: 1 in, 2 out]
        }
        n76 = for {
          tunnel: w134 -> [w154]
          tunnel: string[] ["AI.ini", "AO.ini", "DI.ini", "DO.ini"] -> [w151] mode=indexing
          tunnel: [w148] -> w130 mode=indexing
          tunnel: [w147] -> w132
          n77 = call "Instrument Address.vi"("Command"=Instrument_Address_Command."Init", "error in (no error)"=w154, "name or relative path"=w151) -> ("error out"=w153:errorcluster, "path_out"=w152:path)  [unwired: 6 in, 1 out]
          n78 = call "Instrument Address.vi"("Command"=Instrument_Address_Command."Read", "error in (no error)"=w153, "path_in"=w152) -> ("error out"=w147:errorcluster, "Instrument Parameter"=w150:string[][])  [unwired: 6 in, 1 out]
          n79 = Index Array(array=w150, index (col)=1 ("disabled index (col)")) -> (element=w148:string[])  [unwired: 1 in]
        }
        n80 = Index Array(array=w130, index (row)=1) -> (element=w129:string[])  [unwired: 1 in]
        n81 = control-ref of="AO Name"() -> (w131:refnum<vi>)
        n82 = call "Trim Empty Value.vi"("Data In"=w129) -> ("Data Out"=w128:string[])  [unwired: 10 in]
        n83 = property class="CmbBox"(reference=w131, error in=w132, "Strings[]"=w128) -> (error out=w126:errorcluster)  [unwired: 1 out]
        n84 = call "REQ DC Parameter.vi"("error in"=w126) -> ("error out"=w124:errorcluster)  [unwired: 10 in]
        n85 = Array To Cluster(array=w135) -> (cluster=w141:T31)
        n86 = Bundle By Name(cluster=w145, "Connection?"=w141, "Inst Connected"=w125) -> (w142:T18)
        n87 = property on="CAN Monitor" class="Tbl (strict)"(error in=w124, "Column Headers[]"=string[] ["Timestamp", "Data", "ID", "Type", "Extended?", "Echo?"]) -> (error out=w122:errorcluster)  [unwired: 1 in, 1 out]
      }
      frame "Main" {
        n88 = event shown="[6] \"Digital Output\": Value Change" {
          selector: _ -> [_ _ _ _ _ _ _ _ _ _ _ _ _]
          dyn-events: _ -> [_ _ _ _ _ _ _ _ _ _ _ _ _]
          timeout: -1 -> [_ _ _ _ _ _ _ _ _ _ _ _ _]
          tunnel: w167 -> [w170 w177 w206 w212 w239 w258 w277 w288 w325 w333 w342 w358 w374]
          tunnel: w166 -> [w169 w178 w209 w214 w241 w260 w282 w291 w327 w331 w344 w361 w373]
          tunnel: [w169 w178 w209 w214 w241 w260 w282 w291 w327 w331 w344 w361 w373] -> w165
          tunnel: [Maintenance_command."Main" Maintenance_command."Main" Maintenance_command."Main" Maintenance_command."Main" Maintenance_command."Main" Maintenance_command."Main" Maintenance_command."Main" Maintenance_command."Main" Maintenance_command."Main" Maintenance_command."Main" Maintenance_command."Main" Maintenance_command."Main" Maintenance_command."Close"] -> w164
          tunnel: [w170 w175 _ w211 w238 w257 w272 w287 w322 w332 w340 w357 w374] -> w163
          event Timeout {
            n89 = event-data() -> ()  [unwired: 1 in, 3 out]
          }
          event "DC Apply Command": Value Change {
            n90 = event-data() -> ()  [unwired: 1 in, 6 out]
            n91 = case shown="\"Set Voltage\", Default" "DC PWS Command" {
              tunnel: w177 -> [w184 w189 w190 w192 w195 w204]
              tunnel: [w181 w188 w190 w191 w194 w200] -> w175
              tunnel: "Data In" -> [w180 w187 _ _ _ _]
              tunnel: [_ _ _ _ w193 w199] -> w172
              frame "Set Voltage", Default {
                n92 = Bundle By Name(cluster=T24 {"Address"=0.0, "Voltage Level"=0.0, "Enable Output"=FALSE} ("Output Setting"), "Voltage Level"=w180, "Enable Output"=TRUE) -> (w182:T24)
                n93 = call "REQ Configure Output.vi"("error in"=w184, "Output Setting"=w182) -> ("error out"=w181:errorcluster)  [unwired: 9 in]
              }
              frame "Set Current" {
                n94 = Bundle By Name(cluster=cluster{"Address":dbl, "Current Limit":dbl} {"Address"=0.0, "Current Limit"=0.0} ("Current Limit Setting"), "Current Limit"=w187) -> (w185:cluster{"Address":dbl, "Current Limit":dbl})
                n95 = call "REQ Config Current Limit.vi"("error in"=w189, "Current Limit Setting"=w185) -> ("error out"=w188:errorcluster)  [unwired: 9 in]
              }
              frame "Set Power" {
              }
              frame "DC Parameter" {
                n96 = call "REQ DC Parameter.vi"("error in"=w192) -> ("error out"=w191:errorcluster)  [unwired: 10 in]
              }
              frame "Measure Current" {
                n97 = Bundle By Name(cluster=T25 {"Meas Command"=enum."Voltage", "Address"=0.0} ("Meas Parameter"), "Meas Command"=enum16{"Voltage", "Current", "Power"}."Current") -> (w197:T25)
                n98 = call "REQ Measurement.vi"("error in"=w195, "Meas Parameter"=w197) -> ("error out"=w194:errorcluster, "Value"=w193:dbl)  [unwired: 7 in, 1 out]
              }
              frame "Measure Voltage" {
                n99 = Bundle By Name(cluster=T25 {"Meas Command"=enum."Voltage", "Address"=0.0} ("Meas Parameter"), "Meas Command"=enum16{"Voltage", "Current", "Power"}."Voltage") -> (w202:T25)
                n100 = call "REQ Measurement.vi"("error in"=w204, "Meas Parameter"=w202) -> ("error out"=w200:errorcluster, "Value"=w199:dbl)  [unwired: 7 in, 1 out]
              }
            }
            "Data Out" <- w172
          }
          event "DMM Control": Value Change {
            n101 = event-data() -> ()  [unwired: 1 in, 2 out]
            n102 = Unbundle By Name("DMM Control") -> ("DMM Command"=w205:T32)
            n103 = case shown="\"DC Voltage\", Default" w205 {
              tunnel: w206 -> [_ _ _ _]
              frame "DC Voltage", Default {
              }
              frame "AC Voltage" {
              }
              frame "2 Wire Resistance" {
              }
              frame "Continuity" {
              }
            }
          }
          event "FGen_Apply Command": Value Change {
            n104 = event-data() -> ()  [unwired: 1 in, 6 out]
            n105 = case shown="\"Standad Waveform\", Default" "Input Command" {
              tunnel: w212 -> [w225 w235]
              tunnel: [w224 w234] -> w211
              frame "Standad Waveform", Default {
                n106 = Type Cast(type=u16 0 ("Unit (0: Vpp)"), x="Unit (0: Vpp)") -> (*(type *) &x=w215:u16)
                n107 = Bundle By Name(cluster=T26 {"Waveform Function (1: Sine)"=1, "Frequency (1000 Hz)"=1000.0, "Amplitude (1)"=1.0, "Unit (0: Vpp)"=0, "DC Offset (0.00 V)"=0.0} ("Std Waveform Setting"), "Waveform Function (1: Sine)"="Function", "Frequency (1000 Hz)"="Frequency(1000 Hz)", "Amplitude (1)"="Amplitude", "Unit (0: Vpp)"=w215, "DC Offset (0.00 V)"="DC Offset (V)") -> (w222:T26)
                n108 = call "REQ Config Std Waveform.vi"("error in"=w225, "Std Waveform Setting"=w222) -> ("error out"=w224:errorcluster)  [unwired: 9 in]
              }
              frame "Frequency Sweep" {
                n109 = Type Cast(type=u16 0 ("Sweep Spacing (0: Linear)"), x="Sweep Spacing") -> (*(type *) &x=w230:u16)
                n110 = Bundle By Name(cluster=T27 {"Sweep Spacing (0: Linear)"=0, "Sweep Time (1.00 s)"=1.0, "Stop  Frequency (1000.0 Hz)"=1000.0, "Start Frequency (100.0 Hz)"=100.0, "Enable/Disable Freq Sweep"=FALSE} ("Freq Sweep Setting"), "Sweep Spacing (0: Linear)"=w230, "Sweep Time (1.00 s)"="Sweep Time(Sec)", "Start Frequency (100.0 Hz)"="Start Freq(Hz)", "Stop  Frequency (1000.0 Hz)"="Stop Freq(Hz)") -> (w226:T27)
                n111 = call "REQ Config Freq Sweep.vi"("error in"=w235, "Freq Sweep Setting"=w226) -> ("error out"=w234:errorcluster)  [unwired: 9 in]
              }
            }
          }
          event "ESPEC Apply Command": Value Change {
            n112 = event-data() -> ()  [unwired: 1 in, 2 out]
            n113 = case shown="\"Acquire Data\"" "Meas Command" {
              tunnel: w239 -> [w244 w247 w249 w252 w253 w255]
              tunnel: [w243 w246 w251 w252 w253 w254] -> w238
              tunnel: "ESPEC Apply Command" -> [_ _ w250 _ _ _]
              frame "Output On" {
                n114 = call "REQ Enable Output.vi"("error in"=w244, "Enable Output"=TRUE) -> ("error out"=w243:errorcluster)  [unwired: 9 in]
              }
              frame "Output Off" {
                n115 = call "REQ Enable Output.vi"("error in"=w247, "Enable Output"=FALSE) -> ("error out"=w246:errorcluster)  [unwired: 9 in]
              }
              frame "Acquire Data" {
                n116 = call "REQ Program Status.vi"("error in"=w249) -> ("error out"=w248:errorcluster)  [unwired: 10 in]
                n117 = call "REQ Acquire Data.vi"("error in"=w248, "Acquire Data"=w250) -> ("error out"=w251:errorcluster)  [unwired: 9 in]
              }
              frame "Start Log Data" {
              }
              frame "Stop Log Data" {
              }
              frame "Program Status" {
                n118 = call "REQ Program Status.vi"("error in"=w255) -> ("error out"=w254:errorcluster)  [unwired: 10 in]
              }
            }
          }
          event "Scope Apply Command": Value Change {
            n119 = event-data() -> ()  [unwired: 1 in, 6 out]
            n120 = case shown="\"Acquire Waveform\"" "Scope Command" {
              tunnel: w258 -> [w262 w264 w269 w271]
              tunnel: [w261 w263 w268 w270] -> w257
              frame "Auto Setup", Default {
                n121 = call "REQ Auto setup.vi"("error in"=w262) -> ("error out"=w261:errorcluster)  [unwired: 10 in]
              }
              frame "Config DVM" {
                n122 = call "REQ Configure DVM.vi"("error in"=w264) -> ("error out"=w263:errorcluster)  [unwired: 10 in]
              }
              frame "Config Channel" {
                n123 = Bundle By Name(cluster=T28 {"Channel Name (0: Channel 1)"=0, "Coupling (1: DC)"=1, "Vertical Offset (0.0)"=0.0, "Vertical Range (40.0 V)"=40.0, "Probe Attenuation (1.0)"=1.0, "Enable Channel (T: Enable)"=TRUE, "Impedance (0: 1 MOhm)"=0, "Vertical Scale (5.0 V)"=5.0, "Vertical Setting (1: Vertical Range)"=1} ("Channel Setting"), "Channel Name (0: Channel 1)"="Scope Channel") -> (w266:T28)
                n124 = call "REQ Channel Setting.vi"("error in"=w269, "Channel Setting"=w266) -> ("error out"=w268:errorcluster)  [unwired: 9 in]
              }
              frame "Acquire Waveform" {
                n125 = call "REQ Acq Waveform.vi"("error in"=w271) -> ("error out"=w270:errorcluster)  [unwired: 10 in]
              }
            }
          }
          event "Digital Output": Value Change {
            n126 = event-data() -> ()  [unwired: 1 in, 6 out]
            n127 = call <vilib>:"Read Grouped Tags.vi"("error in (no error)"=w277, "Group"="6515_Digital Output") -> ("error out"=w274:errorcluster, "Data"=w279:T20)  [unwired: 8 in]
            n128 = Unbundle By Name(w279) -> ("Boolean"=w276:bool[])
            n129 = Cluster To Array(cluster="Digital Output") -> (array=w275:bool[])
            n130 = Replace Array Subset(array=w276, new element=w275) -> (w273:bool[])  [unwired: 1 in]
            n131 = call "REQ Write DO.vi"("error in"=w274, "DO Value"=w273) -> ("error out"=w272:errorcluster)  [unwired: 9 in]
          }
          event "NI DAQ Control.Apply Command": Value Change {
            n132 = event-data() -> ()  [unwired: 1 in, 6 out]
            n133 = Unbundle By Name("NI DAQ Control") -> ("NI DAQ Command"=w289:T33, "Sampling rate"=w286:dbl, "AO Name"=w285:string, "AO Data In"=w284:dbl, "Apply Command"=w283:bool)
            n134 = case shown="\"Write AO\"" w289 {
              tunnel: w288 -> [w295 w298 w301 w303 w307 w309 w317 w321]
              tunnel: [w294 w297 w300 w302 w305 w308 w316 w320] -> w287
              tunnel: w286 -> [_ _ _ _ _ _ w314 _]
              tunnel: w285 -> [_ _ _ _ _ _ _ w319]
              tunnel: w284 -> [_ _ _ _ _ _ _ w318]
              tunnel: w283 -> [_ _ _ _ _ _ _ _]
              frame "Acquire AI", Default {
                n135 = call "REQ Acquire AI.vi"("error in"=w295, "Acquire AI"=TRUE) -> ("error out"=w294:errorcluster)  [unwired: 9 in]
              }
              frame "Log Data" {
                n136 = call "REQ Log Data.vi"("error in"=w298, "Log Data"=TRUE) -> ("error out"=w297:errorcluster)  [unwired: 9 in]
              }
              frame "Stop Log Data" {
                n137 = call "REQ Log Data.vi"("error in"=w301, "Log Data"=FALSE) -> ("error out"=w300:errorcluster)  [unwired: 9 in]
              }
              frame "Stop AI" {
                n138 = call "REQ Acquire AI.vi"("error in"=w303, "Acquire AI"=FALSE) -> ("error out"=w302:errorcluster)  [unwired: 9 in]
              }
              frame "Acquire DI" {
                n139 = call "REQ Acquire DI.vi"("error in"=w307, "Acq DI"=TRUE) -> ("error out"=w305:errorcluster)  [unwired: 9 in]
              }
              frame "Stop DI" {
                n140 = call "REQ Acquire DI.vi"("error in"=w309, "Acq DI"=FALSE) -> ("error out"=w308:errorcluster)  [unwired: 9 in]
              }
              frame "Update Rate" {
                n141 = Divide(x=w314, y=10.0) -> (x/y=w312:dbl)
                n142 = Bundle By Name(cluster=T29 {"rate"=1000.0, "samples per channel"=1000, "sample mode"=10123} ("Timing Parameter"), "rate"=w314, "samples per channel"=w312) -> (w311:T29)
                n143 = call "REQ Update Sample Rate.vi"("error in"=w317, "Timing Parameter"=w311) -> ("error out"=w316:errorcluster)  [unwired: 9 in]
              }
              frame "Write AO" {
                n144 = call "REQ Write AO Data.vi"("error in"=w321, "Data"=w318, "AO Name"=w319) -> ("error out"=w320:errorcluster)  [unwired: 8 in]
              }
            }
          }
          event "DIO Apply Comm": Value Change {
            n145 = event-data() -> ()  [unwired: 1 in, 6 out]
            n146 = case shown="\"Acquire DI\", Default" "NI DAQ Command" {
              tunnel: [TRUE FALSE] -> w323
              frame "Acquire DI", Default {
              }
              frame "Stop DI" {
              }
            }
            n147 = call "REQ Acq DI.vi"("error in"=w325, "Acq DI"=w323) -> ("error out"=w322:errorcluster)  [unwired: 9 in]
          }
          event "View Data": Value Change {
            n148 = event-data() -> ()  [unwired: 1 in, 6 out]
            n149 = call "Start Module.vi"("error in"=w333) -> ("error out"=w334:errorcluster, "Wait for Event Sync?"=w335:bool, "Module ID"=w336:i32)  [unwired: 7 in, 1 out]
            n150 = call "Synchronize Module Events.vi"("error in"=w334, "Wait for Event Sync?"=w335, "Module ID in"=w336) -> ("error out"=w337:errorcluster, "Module ID out"=w339:i32)  [unwired: 7 in]
            n151 = call "REQ Initialize Selector.vi"("error in"=w337, "Module ID"=w339) -> ("error out"=w338:errorcluster)  [unwired: 9 in]
            n152 = call "Show Panel.vi"("error in (no error)"=w338, "Module ID"=w339) -> ("error out"=w332:errorcluster)  [unwired: 9 in]
          }
          event "CAN Command": Value Change {
            n153 = event-data() -> ()  [unwired: 1 in, 6 out]
            n154 = case shown="\"Stop Logging Data\"" "NI CAN Command" {
              tunnel: w342 -> [w347 w350 w353 w355 _]
              tunnel: [w346 w349 w352 w354 _] -> w340
              frame "Read CAN Data", Default {
                n155 = call "REQ CAN Data.vi"("error in"=w347, "CAN Read?"=FALSE) -> ("error out"=w346:errorcluster)  [unwired: 9 in]
              }
              frame "Write CAN Data" {
                n156 = call "REQ Write CAN Frame.vi"("error in"=w350, "data"="CAN Frame") -> ("error out"=w349:errorcluster)  [unwired: 9 in]
              }
              frame "Start Logging Data" {
                n157 = call "REQ Start Logging.vi"("error in"=w353, "Start Logging?"=TRUE) -> ("error out"=w352:errorcluster)  [unwired: 9 in]
              }
              frame "Stop Logging Data" {
                n158 = call "REQ Start Logging.vi"("error in"=w355, "Start Logging?"=FALSE) -> ("error out"=w354:errorcluster)  [unwired: 9 in]
              }
              frame "Set Baudrate" {
              }
            }
          }
          event "Serial Apply Command": Value Change {
            n159 = event-data() -> ()  [unwired: 1 in, 6 out]
            n160 = case shown="\"Stop Logging\"" "Serial Command" {
              tunnel: w358 -> [w364 w366 w369 w371]
              tunnel: [w363 w365 w368 w370] -> w357
              frame "Write Data", Default {
                n161 = call "REQ Write Command.vi"("error in"=w364, "Command?"="Command") -> ("error out"=w363:errorcluster)  [unwired: 9 in]
              }
              frame "Acquire Data" {
                n162 = call "REQ Acquire Data.vi"("error in"=w366) -> ("error out"=w365:errorcluster)  [unwired: 10 in]
              }
              frame "Start Logging" {
                n163 = call "REQ Start Logging.vi"("error in"=w369, "Start Logging?"=TRUE) -> ("error out"=w368:errorcluster)  [unwired: 9 in]
              }
              frame "Stop Logging" {
                n164 = call "REQ Start Logging.vi"("error in"=w371, "Start Logging?"=FALSE) -> ("error out"=w370:errorcluster)  [unwired: 9 in]
              }
            }
          }
          event "Exit": Value Change {
            n165 = event-data() -> ()  [unwired: 1 in, 6 out]
          }
        }
      }
      frame "Close" {
        n166 = case shown="True" w382 {
          tunnel: w383 -> [w388 w390]
          tunnel: [w387 w389] -> w379
          frame False {
            n167 = call "Stop Module.vi"("error in"=w388) -> ("error out"=w387:errorcluster)  [unwired: 10 in]
          }
          frame True {
            n168 = call "REQ UI Title.vi"("error in"=w390, "UI Title"="Dashboard" ("ATE Title")) -> ("error out"=w391:errorcluster)  [unwired: 9 in]
            n169 = call "Insert Plugin VI.vi"("VI Name"=VI_Name."Dashboard", "error in (no error)"=w391) -> ("error out"=w389:errorcluster)  [unwired: 9 in]
          }
        }
        n170 = call <vilib>:"Read Grouped Tags.vi"("error in (no error)"=w379, "Group"="6515_Digital Output") -> ("error out"=w377:errorcluster, "Data"=w380:T20)  [unwired: 8 in]
        n171 = Unbundle By Name(w380) -> ("Boolean"=w378:bool[])
        n172 = call "REQ Write DO.vi"("error in"=w377, "DO Value"=w378) -> ("error out"=w376:errorcluster)  [unwired: 9 in]
      }
    }
  }
  n173 = while {
    tunnel: w1 -> [w395]
    tunnel: [w394] -> _
    stop <- w397 stop-if-true
    n174 = event shown="[0] Timeout" {
      selector: _ -> [_ _]
      dyn-events: _ -> [_ _]
      timeout: 100 -> [_ _]
      tunnel: [_ TRUE] -> w397
      tunnel: w395 -> [_ w400]
      tunnel: [_ w398] -> w394
      event Timeout {
        n175 = event-data() -> ()  [unwired: 1 in, 3 out]
      }
      event "Exit": Value Change {
        n176 = event-data() -> ()  [unwired: 1 in, 1 out]
        n177 = call <vilib>:"Read Grouped Tags.vi"("error in (no error)"=w400, "Group"="DMM Parameter") -> ("error out"=w398:errorcluster, "Data"=w402:T20)  [unwired: 8 in]
        n178 = Unbundle By Name(w402) -> ("Double"=w399:dbl[])
        n179 = Index Array(array=w399) -> ()  [unwired: 3 in, 3 out]
      }
    }
  }
  n180 = while {
    tunnel: w1 -> [w404]
    stop <- w406 stop-if-true
    n181 = event shown="[0] Timeout" {
      selector: _ -> [_ _]
      dyn-events: _ -> [_ _]
      timeout: 100 -> [_ _]
      tunnel: [_ TRUE] -> w406
      tunnel: w404 -> [w412 _]
      tunnel: [w408 _] -> _
      event Timeout {
        n182 = event-data() -> ()  [unwired: 1 in, 1 out]
        n183 = call <vilib>:"Read Grouped Tags.vi"("error in (no error)"=w412, "Group"="CAN Frame") -> ("error out"=w408:errorcluster, "Data"=w410:T20)  [unwired: 8 in]
        n184 = Unbundle By Name(w410) -> ("Array of String"=w409:cluster{"String Array":string[]}[])
        n185 = for {
          tunnel: w409 -> [w414] mode=indexing
          tunnel: [w413] -> w407 mode=indexing
          n186 = Unbundle By Name(w414) -> ("String Array"=w413:string[])
        }
        "CAN Monitor" <- w407
      }
      event "Exit": Value Change {
        n187 = event-data() -> ()  [unwired: 1 in, 5 out]
      }
    }
  }
  n188 = while {
    tunnel: w1 -> [w417]
    tunnel: [w416] -> _
    stop <- w418 stop-if-true
    n189 = event shown="[0] Timeout" {
      selector: _ -> [_ _]
      dyn-events: _ -> [_ _]
      timeout: 100 -> [_ _]
      tunnel: [_ TRUE] -> w418
      tunnel: w417 -> [_ w423]
      tunnel: [_ w420] -> w416
      event Timeout {
        n190 = event-data() -> ()  [unwired: 1 in, 3 out]
      }
      event "Exit": Value Change {
        n191 = event-data() -> ()  [unwired: 1 in, 1 out]
        n192 = call <vilib>:"Read Grouped Tags.vi"("error in (no error)"=w423, "Group"="Serial Data") -> ("error out"=w420:errorcluster, "Data"=w421:T20)  [unwired: 8 in]
        n193 = Unbundle By Name(w421) -> ()  [unwired: 1 out]
      }
    }
  }
  n194 = control-ref of="This VI"() -> (w8:refnum<vi>)
  n195 = invoke class="VI" method="FP.Close"(reference=w8, error in=w5) -> (error out=→"error out":errorcluster)  [unwired: 1 in, 2 out]
